vi "host_logging_b2g2.vi"() -> ()   [LabVIEW 2011]
uses:
  <vilib>/addons/database/Connection.llb/Conn ObjectReference.ctl
  Output - Cluster b2g2.ctl
  <vilib>/Platform/TimedLoop/XDataNode/timing_clust.ctl
  <vilib>/Platform/TimedLoop/XDataNode/nitl_modes.ctl
  <vilib>/Platform/TimedLoop/XDataNode/wakeup.ctl
  <vilib>/Platform/TimedLoop/XDataNode/XDataNode.xnode
  <vilib>/Platform/TimedLoop/XDataNode/XDNodeRunTimeDep.lvlib
  <vilib>/addons/database/NI_Database_API.lvlib
panel:
  out "Fehler":errorcluster
  in  "prefix for tables":string(combo)="B2G2"
  in  "interval [s]":u32=10 min=1 step=1
  in  "path":path
  in  "on/off":bool=TRUE
  in  "stop":bool caption="EXIT"
  # "B2G 2 DB Logging"
  # "database logging:"
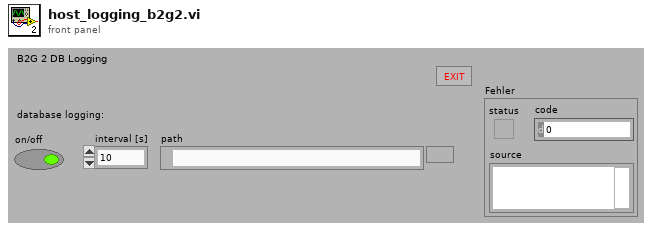
[diagram p1: front panel]
types:
  T1 = typedef "Output - Cluster b2g2.ctl" = cluster{"DFS-1 [dl]":u64, "FS-3 [l]":dbl, "DFS-1 [l/min]":dbl, "DS-1 [bar]":dbl, "V-10 ZU":bool, "V-14 ZU":bool, "FS-1 [l]":dbl, "FS-2 [l]":dbl, "TS-4 [°C]":dbl, "HS-1":bool, "V-13 [%]":u8, "V-15 [%]":u8, "P-4 [%]":u8, "Dosierung":bool, "MR Max Füllstand":bool, "MR Min Füllstand":bool, "Dosiermenge [l]":sgl, "V-14 AUF":bool, "V-10 AUF":bool, "T-1 Max Füllstand":bool, "T-1 Min Füllstand":bool, "T-2 Max Füllstand":bool, "T-2 Min Füllstand":bool, "pHS-1 [pH]":dbl, "P-4 RUN":bool, "V-33 AUF":bool, "V-33 ZU":bool, "V-34 AUF":bool, "V-34 ZU":bool, "P-4 ERR":bool, "TS-5 [°C]":dbl, "V-35 AUF":bool, "V-35 ZU":bool, "P-9 RUN":bool}
  T2 = typedef "NI_Database_API.lvlib/Conn ObjectReference.ctl" = refnum<k1>
  T3 = cluster{"db timing":i64, "DFS-1":u64, "db reference":T2, "P4 RUN":bool, "db":bool, "data refnum":refnum<k21>, "feeding":bool, "feeding start volume":u64, "feeding start time":timestamp, "flashing":bool, "flashing start volume":u64, "flashing start time":timestamp, "V-33":bool, "V-34":bool, "V-15":u8, "V-13":u8, "P4 ERR":bool, "V-14":bool, "V-10":bool, "prefix":string, "V-35":bool, "output cluster reading time":timestamp, "HS1":bool, "P9 RUN":bool}
  T4 = typedef "XDNodeRunTimeDep.lvlib/timing_clust.ctl" = cluster{"Expected End [f-1]":u64, "Actual End [f-1]":u64, "Finished Late? [f-1]":bool, "Expected End [i-1]":u64, "Actual End [i-1]":u64, "Finished Late? [i-1]":bool, "Expected Start [i]":u64, "Actual Start [i]":u64, "Expected Start [f]":u64, "Actual Start [f]":u64, "Source Name":string, "Structure Name":string, "Period":i64, "Deadline":i64, "Offset":i64, "Start":i64, "Priority":i32, "Timeout":i32, "Mode":T5, "Wakeup Reason":T6, "Error":errorcluster, "Source Type":string, "Secondary Source Type":string, "Global End Time":u64, "Global Start Time":u64, "Frame Duration":u64, "Iteration Duration":u64, "Assigned CPU":i32, "I/O Scan Engine Mode":u32}
  T5 = typedef "XDNodeRunTimeDep.lvlib/nitl_modes.ctl" = enum32{"No Change", "Process missed periods, maintain original phase", "Discard missed periods, maintain original phase", "Process missed periods, ignore original phase", "Discard missed periods, ignore original phase"}
  T6 = typedef "XDNodeRunTimeDep.lvlib/wakeup.ctl" = enum32{"Normal", "Aborted", "Asynchronous wakeup", "Timing source error", "Timed loop error", "Timeout"}
  T7 = enum32{"invalid app kind", "Development System", "Run Time System", "Student Edition", "Embedded LabVIEW", "Evaluation", "Custom"}
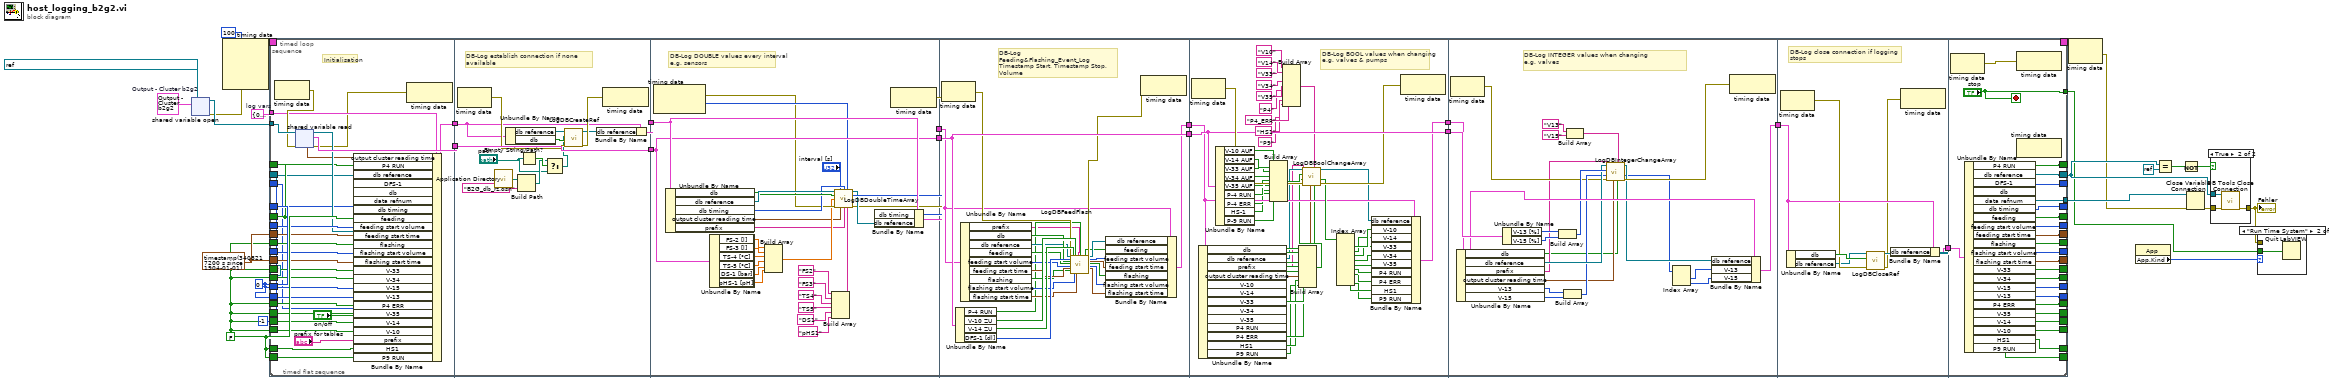
[diagram p0: block diagram]
diagram:
  w14 = T1 {"DFS-1 [dl]"=0, "FS-3 [l]"=0.0, "DFS-1 [l/min]"=0.0, "DS-1 [bar]"=0.0, "V-10 ZU"=FALSE, "V-14 ZU"=FALSE, "FS-1 [l]"=0.0, "FS-2 [l]"=0.0, "TS-4 [°C]"=0.0, "HS-1"=FALSE, "V-13 [%]"=0, "V-15 [%]"=0, "P-4 [%]"=0, "Dosierung"=FALSE, "MR Max Füllstand"=FALSE, "MR Min Füllstand"=FALSE, "Dosiermenge [l]"=0.0, "V-14 AUF"=FALSE, "V-10 AUF"=FALSE, "T-1 Max Füllstand"=FALSE, "T-1 Min Füllstand"=FALSE, "T-2 Max Füllstand"=FALSE, "T-2 Min Füllstand"=FALSE, "pHS-1 [pH]"=0.0, "P-4 RUN"=FALSE, "V-33 AUF"=FALSE, "V-33 ZU"=FALSE, "V-34 AUF"=FALSE, "V-34 ZU"=FALSE, "P-4 ERR"=FALSE, "TS-5 [°C]"=0.0, "V-35 AUF"=FALSE, "V-35 ZU"=FALSE, "P-9 RUN"=FALSE}  # Output - Cluster b2g2
  w16 = T3 {"db timing"=0, "DFS-1"=0, "db reference"=refnum, "P4 RUN"=FALSE, "db"=FALSE, "data refnum"="ni.var.psp://10.27.40.21/variables - network - RT (separate)/data - network", "feeding"=FALSE, "feeding start volume"=0, "feeding start time"=timestamp(0 s since 1904-01-01), "flashing"=FALSE, "flashing start volume"=0, "flashing start time"=timestamp(0 s since 1904-01-01), "V-33"=FALSE, "V-34"=FALSE, "V-15"=0, "V-13"=0, "P4 ERR"=FALSE, "V-14"=FALSE, "V-10"=FALSE, "prefix"="", "V-35"=FALSE, "output cluster reading time"=timestamp(0 s since 1904-01-01), "HS1"=FALSE, "P9 RUN"=FALSE}  # log vars
  w9 = timestamp(3408217200 s since 1904-01-01) ("Time Stamp")
  w1 = FALSE ("P5")
  w10 = -1
  w8 = i64 0 ("Actual Start [i]")
  n1 = shared-variable-open(refnum<k21> "ni.var.psp://10.27.40.25/variables - b2g2/data - network b2g2" ("output variable"), w14) -> (w15:refnum<k21>, w7:errorcluster)  [unwired: 2 in]
  n2 = node-c288(i64 100 ("Period"), w7) -> (w23:T4)  [unwired: 2 in]
  n3 = timed-loop {
    timing: w23 -> [_]
    timing-out: [_] -> w22
    shift-right: [w66] -> _
    shift-left: w8 -> [w67]
    tunnel: w16 -> [w65]
    shift-right: [w64] -> _
    shift-left: w10 -> [w57]
    shift-right: [w63] -> w17
    shift-left: refnum<k0> refnum -> [w62]
    shift-right: [w61] -> _
    shift-left: w1 -> [w60]
    tunnel: w15 -> [w59]
    tunnel: [w58] -> w12
    shift-right: [w56] -> _
    shift-left: w1 -> [w55]
    shift-right: [w54] -> _
    shift-left: w1 -> [w53]
    shift-right: [w52] -> _
    shift-left: w10 -> [w51]
    shift-right: [w50] -> _
    shift-left: w10 -> [w49]
    shift-right: [w48] -> _
    shift-left: w9 -> [w47]
    shift-right: [w46] -> _
    shift-left: w9 -> [w45]
    shift-right: [w44] -> _
    shift-left: w8 -> [w38]
    shift-right: [w43] -> _
    shift-left: w8 -> [w37]
    shift-right: [w42] -> _
    shift-left: w1 -> [w39]
    shift-right: [w41] -> _
    shift-left: w1 -> [w40]
    shift-right: [w36] -> _
    shift-left: w1 -> [w35]
    shift-right: [w34] -> _
    shift-left: w1 -> [w31]
    shift-right: [w33] -> _
    shift-left: w1 -> [w32]
    shift-right: [w30] -> _
    shift-left: w1 -> [w29]
    tunnel: [w28] -> w3
    shift-right: [w27] -> _
    shift-left: w1 -> [w26]
    shift-right: [w25] -> _
    shift-left: w1 -> [w24]
    stop <- "stop" stop-if-true
    n4 = timed-sequence {
      timing: _ -> [_]
      timing-out: _ -> [_]
      tunnel: w67 -> [w123]
      tunnel: [w122] -> w66
      tunnel: w65 -> [w121]
      tunnel: [w120] -> w64
      tunnel: [w119] -> w63
      tunnel: w62 -> [w118]
      tunnel: [w117] -> w61
      tunnel: w60 -> [w116]
      tunnel: w59 -> [w111]
      tunnel: [w110] -> w58
      tunnel: w57 -> [w109]
      tunnel: [w106] -> w56
      tunnel: w55 -> [w105]
      tunnel: [w104] -> w54
      tunnel: w53 -> [w103]
      tunnel: [w102] -> w52
      tunnel: w51 -> [w101]
      tunnel: [w100] -> w50
      tunnel: w49 -> [w99]
      tunnel: [w98] -> w48
      tunnel: w47 -> [w97]
      tunnel: [w96] -> w46
      tunnel: w45 -> [w95]
      tunnel: [w92] -> w44
      tunnel: [w91] -> w43
      tunnel: [w90] -> w42
      tunnel: [w89] -> w41
      tunnel: w40 -> [w88]
      tunnel: w39 -> [w87]
      tunnel: w38 -> [w86]
      tunnel: w37 -> [w85]
      tunnel: [w81] -> w36
      tunnel: w35 -> [w80]
      tunnel: [w79] -> w34
      tunnel: [w78] -> w33
      tunnel: w32 -> [w77]
      tunnel: w31 -> [w76]
      tunnel: [w75] -> w30
      tunnel: w29 -> [w74]
      tunnel: [w72] -> w28
      tunnel: [w71] -> w27
      tunnel: w26 -> [w70]
      tunnel: [w69] -> w25
      tunnel: w24 -> [w68]
      n5 = timed-flat-sequence {
        tunnel: w123 -> [w129]
        tunnel: [w151] -> w115
        tunnel: w121 -> [w137]
        tunnel: [w136] -> w113
        tunnel: w118 -> [w127]
        tunnel: w116 -> [w138]
        tunnel: w111 -> [w153]
        tunnel: w109 -> [w128]
        tunnel: w105 -> [w141]
        tunnel: w103 -> [w144]
        tunnel: w101 -> [w142]
        tunnel: w99 -> [w145]
        tunnel: w97 -> [w146]
        tunnel: w95 -> [w143]
        tunnel: w88 -> [w147]
        tunnel: w87 -> [w148]
        tunnel: w86 -> [w149]
        tunnel: w85 -> [w150]
        tunnel: w80 -> [w135]
        tunnel: w77 -> [w133]
        tunnel: w76 -> [w134]
        tunnel: w74 -> [w131]
        tunnel: w70 -> [w125]
        tunnel: w68 -> [w124]
        tunnel: w115 -> [w172]
        tunnel: [w172] -> w114
        tunnel: w113 -> [w168]
        tunnel: [w167] -> w112
        tunnel: w114 -> [w191]
        tunnel: [w191] -> w108
        tunnel: w112 -> [w204]
        tunnel: [w205] -> w107
        tunnel: w108 -> [w236]
        tunnel: [w236] -> w94
        tunnel: w107 -> [w224]
        tunnel: [w230] -> w93
        tunnel: w94 -> [w290]
        tunnel: [w290] -> w84
        tunnel: w93 -> [w274]
        tunnel: [w275] -> w83
        tunnel: w84 -> [w317]
        tunnel: w83 -> [w314]
        tunnel: [w318] -> w82
        tunnel: w82 -> [w329]
        tunnel: [w324] -> w73
        tunnel: [w341] -> w122
        tunnel: [w340] -> w120
        tunnel: [w339] -> w119
        tunnel: [w358] -> w117
        tunnel: [w357] -> w110
        tunnel: [w356] -> w106
        tunnel: [w353] -> w104
        tunnel: [w355] -> w102
        tunnel: [w352] -> w100
        tunnel: [w351] -> w98
        tunnel: [w354] -> w96
        tunnel: [w348] -> w92
        tunnel: [w347] -> w91
        tunnel: [w349] -> w90
        tunnel: [w350] -> w89
        tunnel: [w346] -> w81
        tunnel: [w345] -> w79
        tunnel: [w344] -> w78
        tunnel: [w343] -> w75
        tunnel: w73 -> [w342]
        tunnel: ["stop"] -> w72
        tunnel: [w337] -> w71
        tunnel: [w336] -> w69
        frame #0 {
          # "Initialisation"
          n6 = node-c288() -> (w152:errorcluster)  [unwired: 1 in]
          n7 = shared-variable-read(w153, w152) -> (w140:refnum<k21>, w130:errorcluster, w151:T1, w126:timestamp)
          n8 = Bundle By Name(cluster=w137, "output cluster reading time"=w126, "P4 RUN"=w138, "db reference"=w127, "DFS-1"=w128, "db"="on/off", "data refnum"=w140, "db timing"=w129, "feeding"=w141, "feeding start volume"=w142, "feeding start time"=w143, "flashing"=w144, "flashing start volume"=w145, "flashing start time"=w146, "V-33"=w147, "V-34"=w148, "V-15"=w149, "V-13"=w150, "P4 ERR"=w135, "V-35"=w131, "V-14"=w134, "V-10"=w133, "prefix"="prefix for tables", "HS1"=w125, "P9 RUN"=w124) -> (w136:T3)
          n9 = node-c288(w130) -> ()  [unwired: 1 out]
        }
        frame #1 {
          # "DB-Log establish connection if none available"
          n10 = node-c288() -> (w170:errorcluster)  [unwired: 1 in]
          n11 = call <vilib>:"Application Directory.vi"() -> ("Application Directory"=w162:path)
          n12 = Unbundle By Name(w168) -> ("db reference"=w171:T2, "db"=w165:bool)
          n13 = Build Path(base path=w162, name or relative path="B2G_db_rz.dsn" ("Name of ini file 2")) -> (appended path=w163:path)
          n14 = Empty String/Path?(string/path="path") -> (empty?=w164:bool)
          n15 = Select(t=w163, s=w164, f="path") -> (s? t:f=w159:path)
          n16 = call "LogDBCreateRef.vi"("error in (no error)"=w170, "db"=w165, "Pfad in"=w159, "Refnum in"=w171) -> ("error out"=w169:errorcluster, "Refnum out"=w166:T2)  [unwired: 6 in]
          n17 = Bundle By Name(cluster=w168, "db reference"=w166) -> (w167:T3)
          n18 = node-c288(w169) -> ()  [unwired: 1 out]
        }
        frame #2 {
          # "DB-Log DOUBLE values every interval\ne.g. sensors"
          n19 = node-c288() -> (w182:errorcluster, w186:i64)  [unwired: 1 in]
          n20 = Unbundle By Name(w204) -> ("db"=w189:bool, "db reference"=w190:T2, "db timing"=w188:i64, "output cluster reading time"=w178:timestamp, "prefix"=w179:string)
          n21 = Unbundle By Name(w191) -> ("FS-2 [l]"=w192:dbl, "FS-3 [l]"=w193:dbl, "TS-4 [°C]"=w194:dbl, "TS-5 [°C]"=w195:dbl, "DS-1 [bar]"=w196:dbl, "pHS-1 [pH]"=w197:dbl)
          n22 = Build Array(w192, w193, w194, w195, w196, w197) -> (w181:dbl[])
          n23 = Build Array("FS2" ("table"), "FS3" ("table"), "TS4" ("table"), "TS5" ("table"), "DS1" ("table"), "pHS1" ("table")) -> (w180:string[])
          n24 = call "LogDBDoubleTimeArray.vi"("Refnum in"=w190, "db Interval [s]"="interval [s]", "db timing"=w188, "Actual Start [f] in"=w186, "db"=w189, "values"=w181, "error in (no error)"=w182, "Time Stamp"=w178, "prefix"=w179, "names"=w180) -> ("Refnum out"=w184:T2, "Actual Start [f] out"=w185:i64, "error out"=w183:errorcluster)  [unwired: 3 in]
          n25 = Bundle By Name(cluster=w204, "db timing"=w185, "db reference"=w184) -> (w205:T3)
          n26 = node-c288(w183) -> ()  [unwired: 1 out]
        }
        frame #3 {
          # "DB-Log\nFeeding&Flashing_Event_Log\nTimestamp Start, Timestamp Stop, Volume"
          n27 = node-c288() -> (w232:errorcluster)  [unwired: 1 in]
          n28 = Unbundle By Name(w236) -> ("P-4 RUN"=w213:bool, "V-10 ZU"=w234:bool, "V-14 ZU"=w233:bool, "DFS-1 [dl]"=w235:u64)
          n29 = Unbundle By Name(w224) -> ("prefix"=w212:string, "db"=w227:bool, "db reference"=w226:T2, "feeding"=w214:bool, "feeding start volume"=w225:u64, "feeding start time"=w223:timestamp, "flashing"=w215:bool, "flashing start volume"=w217:u64, "flashing start time"=w216:timestamp)
          n30 = call "LogDBFeedFlash.vi"("Refnum in"=w226, "value volume [dl]"=w235, "enable"=w227, "feeding"=w214, "feeding start volume"=w225, "feeding start time"=w223, "flashing"=w215, "error in"=w232, "valve t-2 close"=w233, "flashing start volume"=w217, "valve t-1 close"=w234, "flashing start time"=w216, "prefix"=w212, "Pump"=w213) -> ("feeding"=w228:bool, "Refnum out"=w229:T2, "feeding start volume"=w221:u64, "feeding start time"=w222:timestamp, "flashing"=w219:bool, "flashing start volume"=w218:u64, "flashing start time"=w220:timestamp, "error out"=w231:errorcluster)  [unwired: 6 in]
          n31 = Bundle By Name(cluster=w224, "db reference"=w229, "feeding"=w228, "feeding start volume"=w221, "feeding start time"=w222, "flashing"=w219, "flashing start volume"=w218, "flashing start time"=w220) -> (w230:T3)
          n32 = node-c288(w231) -> ()  [unwired: 1 out]
        }
        frame #4 {
          # "DB-Log BOOL values when changing\ne.g. valves & pumps"
          n33 = node-c288() -> (w291:errorcluster)  [unwired: 1 in]
          n34 = Unbundle By Name(w274) -> ("db"=w252:bool, "db reference"=w263:T2, "prefix"=w262:string, "output cluster reading time"=w261:timestamp, "V-10"=w273:bool, "V-14"=w272:bool, "V-33"=w271:bool, "V-34"=w270:bool, "V-35"=w269:bool, "P4 RUN"=w268:bool, "P4 ERR"=w267:bool, "HS1"=w250:bool, "P9 RUN"=w242:bool)
          n35 = Unbundle By Name(w290) -> ("V-10 AUF"=w289:bool, "V-14 AUF"=w288:bool, "V-33 AUF"=w287:bool, "V-34 AUF"=w286:bool, "V-35 AUF"=w285:bool, "P-4 RUN"=w249:bool, "P-4 ERR"=w248:bool, "HS-1"=w247:bool, "P-9 RUN"=w245:bool)
          n36 = Build Array(w289, w288, w287, w286, w285, w249, w248, w247, w245) -> (w277:bool[])
          n37 = Build Array("V10" ("table"), "V14" ("table"), "V33" ("table"), "V34" ("table"), "V35" ("table"), "P4" ("table"), "P4_ERR" ("table"), "HS1" ("table"), "P9" ("table")) -> (w278:string[])
          n38 = Build Array(w273, w272, w271, w270, w269, w268, w267, w250, w242) -> (w264:bool[])
          n39 = call "LogDBBoolChangeArray.vi"("db"=w252, "names"=w278, "cluster reading time"=w261, "prefix"=w262, "error in (no error)"=w291, "shift reg in"=w264, "values"=w277, "db reference"=w263) -> ("error out"=w279:errorcluster, "shift reg out"=w276:bool[], "db reference out"=w253:T2)  [unwired: 1 in]
          n40 = Index Array(array=w276) -> (element #1=w260:bool, element #2=w259:bool, element #3=w258:bool, element #4=w257:bool, element #5=w256:bool, element #6=w255:bool, element #7=w254:bool, element #8=w251:bool, element #9=w243:bool)  [unwired: 9 in]
          n41 = Bundle By Name(cluster=w274, "db reference"=w253, "V-10"=w260, "V-14"=w259, "V-33"=w258, "V-34"=w257, "V-35"=w256, "P4 RUN"=w255, "P4 ERR"=w254, "HS1"=w251, "P9 RUN"=w243) -> (w275:T3)
          n42 = node-c288(w279) -> ()  [unwired: 1 out]
        }
        frame #5 {
          # "DB-Log INTEGER values when changing\ne.g. valves"
          n43 = node-c288() -> (w305:errorcluster)  [unwired: 1 in]
          n44 = Unbundle By Name(w314) -> ("db"=w297:bool, "db reference"=w309:T2, "prefix"=w298:string, "output cluster reading time"=w299:timestamp, "V-13"=w308:u8, "V-15"=w307:u8)
          n45 = Unbundle By Name(w317) -> ("V-13 [%]"=w312:u8, "V-15 [%]"=w311:u8)
          n46 = Build Array(w312, w311) -> (w310:u8[])
          n47 = Build Array(w308, w307) -> (w306:u8[])
          n48 = Build Array("V13" ("table"), "V15" ("table")) -> (w313:string[])
          n49 = call "LogDBIntegerChangeArray.vi"("db"=w297, "names"=w313, "current time"=w299, "prefix"=w298, "error in (no error)"=w305, "shift reg in"=w306, "values"=w310, "Refnum in"=w309) -> ("error out"=w304:errorcluster, "shift reg out"=w300:u8[], "Refnum out"=w303:T2)  [unwired: 1 in]
          n50 = Index Array(array=w300) -> (element #1=w302:u8, element #2=w301:u8)  [unwired: 2 in]
          n51 = Bundle By Name(cluster=w314, "db reference"=w303, "V-13"=w302, "V-15"=w301) -> (w318:T3)
          n52 = node-c288(w304) -> ()  [unwired: 1 out]
        }
        frame #6 {
          # "DB-Log close connection if logging stops"
          n53 = node-c288() -> (w327:errorcluster)  [unwired: 1 in]
          n54 = Unbundle By Name(w329) -> ("db"=w328:bool, "db reference"=w325:T2)
          n55 = call "LogDBCloseRef.vi"("error in (no error)"=w327, "enable"=w328, "Refnum in"=w325) -> ("error out"=w326:errorcluster, "Refnum out"=w330:T2)  [unwired: 7 in]
          n56 = Bundle By Name(cluster=w329, "db reference"=w330) -> (w324:T3)
          n57 = node-c288(w326) -> ()  [unwired: 1 out]
        }
        frame #7 {
          n58 = node-c288() -> (w359:errorcluster)  [unwired: 1 in]
          n59 = Unbundle By Name(w342) -> ("P4 RUN"=w358:bool, "db reference"=w339:T2, "DFS-1"=w340:u64, "data refnum"=w357:refnum<k21>, "db timing"=w341:i64, "feeding"=w356:bool, "feeding start volume"=w355:u64, "feeding start time"=w354:timestamp, "flashing"=w353:bool, "flashing start volume"=w352:u64, "flashing start time"=w351:timestamp, "V-33"=w350:bool, "V-34"=w349:bool, "V-15"=w348:u8, "V-13"=w347:u8, "P4 ERR"=w346:bool, "V-35"=w343:bool, "V-14"=w345:bool, "V-10"=w344:bool, "HS1"=w337:bool, "P9 RUN"=w336:bool)  [unwired: 1 out]
          n60 = node-c288(w359) -> ()  [unwired: 1 out]
        }
      }
    }
    n61 = node-c288() -> ()  [unwired: 1 in, 1 out]
    n62 = node-c288() -> ()  [unwired: 1 in, 1 out]
  }
  n63 = node-c288(w22) -> (w11:errorcluster)
  n64 = property class="App"() -> ("App.Kind"=w4:T7)  [unwired: 2 in, 2 out]
  n65 = Equal?(x=w17, y=refnum<k0> refnum) -> (x = y?=w20:bool)
  n66 = Not(x=w20) -> (.not. x?=w18:bool)
  n67 = Close Variable Connection(8:w11, 11:w12) -> (0:w6:errorcluster)
  n68 = case shown="True" w18 {
    tunnel: w6 -> [w367 w370]
    tunnel: w17 -> [_ w369]
    tunnel: [w367 w368] -> w2
    frame False {
    }
    frame True {
      n69 = call <vilib>:"DB Tools Close Connection.vi"("error in (no error)"=w370, "connection reference"=w369) -> ("error out"=w368:errorcluster)  [unwired: 5 in]
    }
  }
  "Fehler" <- w2
  n70 = case shown="\"Run Time System\"" w4 {
    tunnel: w3 -> [_ w371 _]
    tunnel: w2 -> [_ _ _]
    frame "invalid app kind", Default {
    }
    frame "Run Time System" {
      n71 = Quit LabVIEW(quit? (T)=w371) -> ()
    }
    frame "Development System" {
    }
  }
